vi "Making a Dark Sky Time Machine Request.vi"() -> ()   [LabVIEW 2017, in "Dark Sky Weather Data for LabVIEW.lvlib"]
doc: "This example makes a Time Machine request to the DarkSky API and interprets the result. A Time Machine request returns the observed (in the past) or forecasted (in the future) hour-by-hour weather and daily weather conditions for a particular date."
uses:
  Dark Sky Weather Data for LabVIEW.lvlib
  Controls/Units Enum.ctl
  Controls/Language Enum.ctl
panel:
  in  "Request Date/Time":timestamp=timestamp(3569396400 s since 1904-01-01)
  out "Current Conditions for Request":string
  out "Timezone of Request":string
  in  "Language":T1=enum."English"
  in  "Units":T2="auto"
  in  "Longitude":dbl=-71.0589 min=-180.0 max=180.0
  in  "Latitude":dbl=42.3601 min=-90.0 max=90.0
  in  "API Key":string
  # "Time Machine Request"
  # "Powered by Dark Sky"
  # "Required Inputs"
  # "Example Response Subset"
  # "The Time Machine request returns a variety of data. Here is an example where you pull out just the timezone of the requested location along with the summary of current conditions for a time in the past. In this example the default values of latitude and longitude coordinates are for Boston, MA, USA, and the default value for Request Date/Time is February 8, 2017 at 6:00 AM local time.\n\nConditions should be snowy at this time in the past.\n\nVisit https://darksky.net/dev/docs\nfor a complete summary of the data returned by Time Machine requests."
  # "Time Machine requests output weather data for a given day including the overall data for the day, data by the hour of that day, and the current data for a specific minute in that day for a given location in longitude and latitude coordinates. These requests can be made for past, current, or future dates.\n\nIn order to make a Time Machine request, you will need an API key and have already determine the longitude and latitude coordinates of the location you are interested in.\n\nNeed an API Key? Visit: https://darksky.net/dev/ and sign up for free! Enter this API key into the API Key input to run this example."
  # "Optional Inputs"
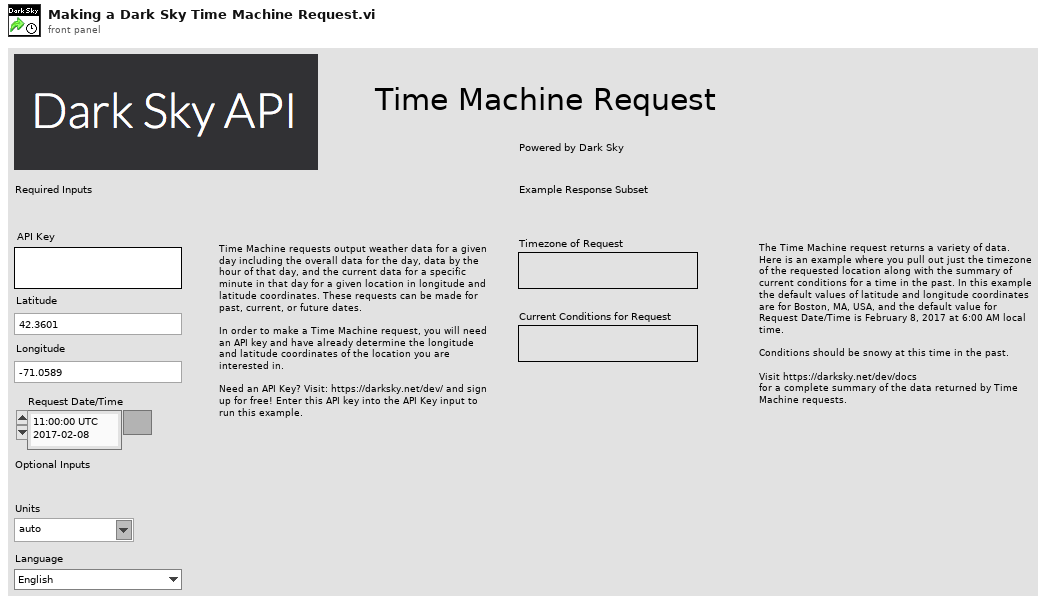
[diagram p1: front panel]
types:
  T1 = typedef "Dark Sky Weather Data for LabVIEW.lvlib/Language Enum.ctl" = enum16{"Arabic", "Azerbaijani", "Belaursian", "Bulgarian", "Bosnian", "Catalan", "Czech", "German", "Greek", "English", "Spanish", "Estonian", "French", "Croatian", "Hungarian", "Indonesian", "Italian", "Icelandic", "Georgian", "Cornish", "Norwegian Bokmal", "Dutch", "Polish", "Portuguese", "Russian", "Slovak", "Slovenian", "Serbian", "Swedish", "Tetum", "Turkish", "Ukrainian", "simplified Chinese", "traditional Chinese"}
  T2 = typedef "Dark Sky Weather Data for LabVIEW.lvlib/Units Enum.ctl" = string
  T3 = typedef "Dark Sky Weather Data for LabVIEW.lvlib/Lat_Lon_TZ.ctl" = cluster{"latitude":dbl, "longitude":dbl, "timezone":string, "offset":dbl}
  T4 = typedef "Dark Sky Weather Data for LabVIEW.lvlib/Forecast Current Data.ctl" = cluster{"currently":cluster{"time":dbl, "summary":string, "icon":string, "nearestStormDistance":dbl, "precipIntensity":dbl, "PrecipIntensityError":dbl, "precipProbability":dbl, "precipType":string, "temperature":dbl, "apparentTemp":dbl, "dewPoint":dbl, "humidity":dbl, "windSpeed":dbl, "windGust":dbl, "windBearing":dbl, "visibility":dbl, "cloudCover":dbl, "pressure":dbl, "ozone":dbl}}
  T5 = cluster{"Lat, Long, Timezone":T3, "Current Data":T4, "Hourly Data":cluster{"hourly":cluster{"summary":string, "icon":string, "data":cluster{"time":dbl, "summary":string, "icon":string, "precipIntensity":dbl, "precipProbability":dbl, "precipType":string, "temperature":dbl, "apparentTemp":dbl, "dewPoint":dbl, "humidity":dbl, "windSpeed":dbl, "windGust":dbl, "windBearing":dbl, "visibility":dbl, "cloudCover":dbl, "pressure":dbl, "ozone":dbl}[]}}, "Daily Data":cluster{"daily":cluster{"data":cluster{"time":dbl, "summary":string, "icon":string, "sunriseTime":dbl, "sunsetTime":dbl, "moonPhase":dbl, "precipIntensity":dbl, "precipIntensityMax":dbl, "precipIntensityMaxTime":dbl, "precipProbability":dbl, "precipType":string, "temperatureMin":dbl, "temperatureMinTime":dbl, "temperatureMax":dbl, "temperatureMaxTime":dbl, "apparentTempMin":dbl, "apparentTempMinTime":dbl, "apparentTempMax":dbl, "apparentTempMaxTime2":dbl, "dewPoint":dbl, "humidity":dbl, "windSpeed":dbl, "windBearing":dbl, "visibility":dbl, "cloudCover":dbl, "pressure":dbl, "ozone":dbl}[]}}}
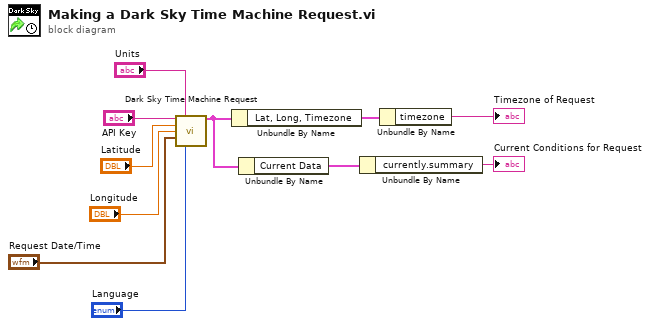
[diagram p0: block diagram]
diagram:
  n1 = call "Dark Sky Time Machine Request.vi"("API Key"="API Key", "Units"="Units", "Latitude"="Latitude", "Longitude"="Longitude", "Time Machine Date/Time"="Request Date/Time", "Language"="Language") -> ("Time Machine Forecast Output"=w3:T5)  [unwired: 8 in, 1 out]
  n2 = Unbundle By Name(w3) -> ("Lat, Long, Timezone"=w5:T3)
  n3 = Unbundle By Name(w3) -> ("Current Data"=w2:T4)
  n4 = Unbundle By Name(w2) -> ("currently.summary"=→"Current Conditions for Request":string)
  n5 = Unbundle By Name(w5) -> ("timezone"=→"Timezone of Request":string)
